vi "Configure.vi"(8 "error in (no error)":errorcluster, 11 "Retiga in":refnum<class "Retiga.lvclass">) -> (0 "error out":errorcluster, 2 "cancelled?":bool, 3 "Retiga out":refnum<class "Retiga.lvclass">)   [LabVIEW 2012, in "Retiga.lvclass"]
doc: "The configure method configures the details for the RabbitMQ connection, the observers and the mapping script.\n\nIn the derived class, make a call to the parent for setting these parameters."
uses:
  Retiga.lvclass
  <vilib>/Utility/miscctls.llb/LVPointTypeDef.ctl
  Retiga.lvclass/Retiga.ctl
  <vilib>/Distrio/Murmex/Murmex/Murmex.lvclass
panel:
  in  "button:call_parent":bool
  in  "button:cancel":bool
  in  "button:ok":bool
  in  "Tab Control":enum32{"Phase comparison", "Camera properties"}(tab)
  in  "stage component":string
  in  "micron equivalent of pixel":dbl[unit]
  in  "max x pixel displacement":dbl
  in  "max pixel discrepancy":dbl
  in  "max y pixel displacement":dbl
  in  "max physical displacement":dbl[unit]
  in  "brightness threshold":sgl
  in  "min physical displacement":dbl[unit]
  in  "temperature":dbl
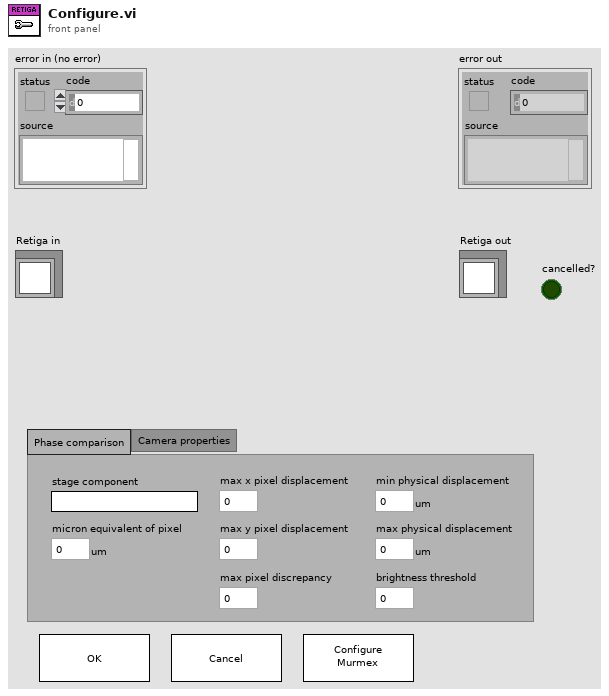
[diagram p1: front panel]
types:
  T1 = typedef "LVPointTypeDef.ctl" = cluster{"Horizontal":i16, "Vertical":i16}
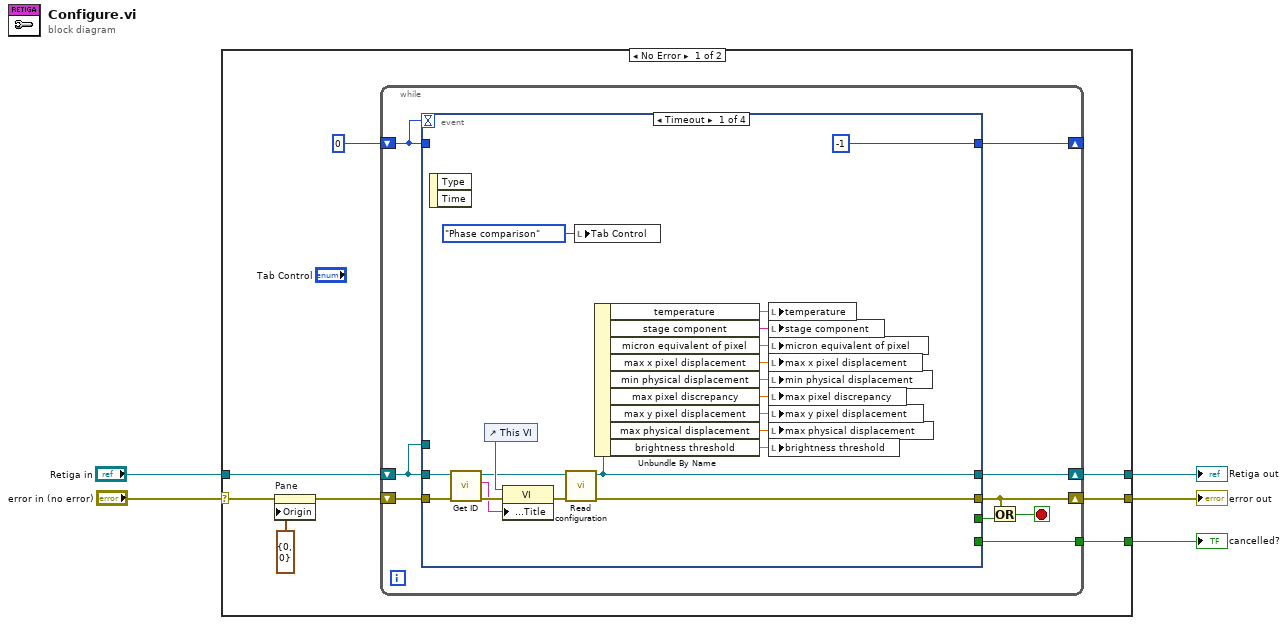
[diagram p0: block diagram]
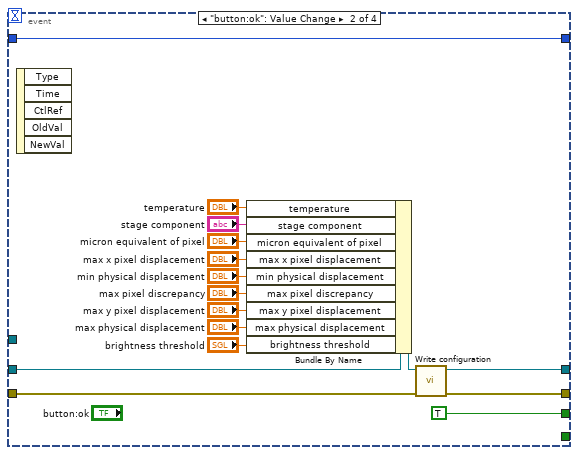
[diagram p2: hidden frame]
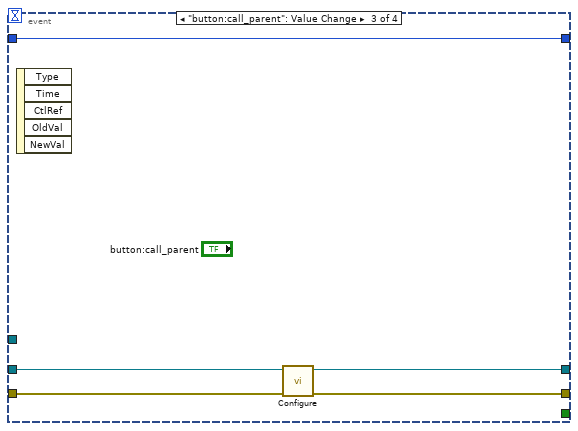
[diagram p3: hidden frame]
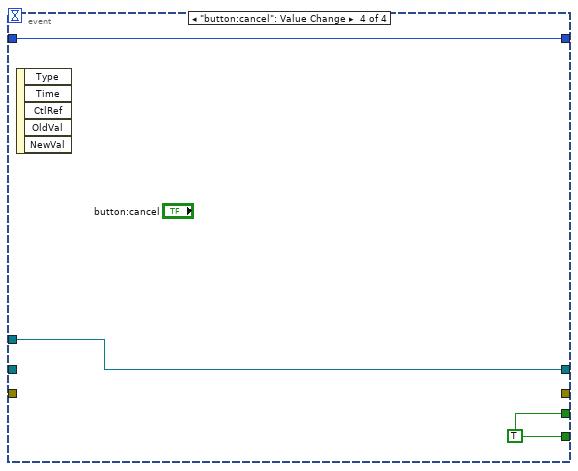
[diagram p4: hidden frame]
diagram:
  n1 = case shown="No Error" "error in (no error)" {
    selector: "error in (no error)" -> [w12 w67]
    tunnel: [w7 w68] -> w4
    tunnel: "Retiga in" -> [w10 w68]
    tunnel: [w8 w67] -> w2
    tunnel: [w6 _] -> w1
    frame No Error {
      n2 = property on="Pane" class="Pane"(error in=w12, "Origin"=T1 {"Horizontal"=0, "Vertical"=0}) -> (error out=w11:errorcluster)  [unwired: 1 in, 1 out]
      n3 = while {
        shift-right: [w16] -> w8
        shift-left: w11 -> [w22]
        shift-right: [w18] -> w7
        shift-left: w10 -> [w21]
        shift-right: [w19] -> _
        shift-left: 0 -> [w20]
        tunnel: [w14] -> w6
        stop <- w15 stop-if-true
        n4 = event shown="[0] Timeout" {
          selector: _ -> [_ _ _ _]
          dyn-events: _ -> [_ _ _ _]
          timeout: w20 -> [_ _ _ _]
          tunnel: w22 -> [w36 w58 w63 _]
          tunnel: w21 -> [w35 w56 w62 _]
          tunnel: w21 -> [_ _ _ w66]
          tunnel: w20 -> [_ w43 w59 w64]
          tunnel: [-1 w43 w59 w64] -> w19
          tunnel: [w33 w57 w60 _] -> w16
          tunnel: [w34 w54 w61 w66] -> w18
          tunnel: [_ TRUE ("y") _ w65] -> w17
          tunnel: [_ _ _ w65] -> w14
          event Timeout {
            n5 = event-data() -> ()  [unwired: 1 in, 2 out]
            n6 = call <vilib>:"Get ID.vi"("error in (no error)"=w36, "Murmex in"=w35) -> ("error out"=w41:errorcluster, "component id"=w37:string, "Murmex out"=w38:refnum<class "Retiga.lvclass">)  [unwired: 7 in]
            n7 = control-ref of="This VI"() -> (w40:refnum<vi>)
            n8 = property class="VI"(reference=w40, error in=w41, "Front Panel.Title"=w37) -> (error out=w39:errorcluster)  [unwired: 1 out]
            n9 = call <vilib>:"Read configuration.vi"("error in (no error)"=w39, "Murmex in"=w38) -> ("error out"=w33:errorcluster, "Murmex out"=w34:refnum<class "Retiga.lvclass">)  [unwired: 7 in, 1 out]
            n10 = local write "Tab Control"(enum32{"Phase comparison", "Camera properties"}."Phase comparison" ("Tab Control")) -> ()
            n11 = Unbundle By Name(w34) -> ("temperature"=w27:dbl, "stage component"=w26:string, "micron equivalent of pixel"=w28:dbl[unit], "max x pixel displacement"=w25:dbl, "min physical displacement"=w30:dbl[unit], "max pixel discrepancy"=w31:dbl, "max y pixel displacement"=w32:dbl, "max physical displacement"=w24:dbl[unit], "brightness threshold"=w29:sgl)
            n12 = local write "temperature"(w27) -> ()
            n13 = local write "stage component"(w26) -> ()
            n14 = local write "micron equivalent of pixel"(w28) -> ()
            n15 = local write "max x pixel displacement"(w25) -> ()
            n16 = local write "min physical displacement"(w30) -> ()
            n17 = local write "max pixel discrepancy"(w31) -> ()
            n18 = local write "max y pixel displacement"(w32) -> ()
            n19 = local write "max physical displacement"(w24) -> ()
            n20 = local write "brightness threshold"(w29) -> ()
          }
          event "button:ok": Value Change {
            n21 = event-data() -> ()  [unwired: 1 in, 5 out]
            n22 = Bundle By Name(cluster=w56, "temperature"="temperature", "stage component"="stage component", "micron equivalent of pixel"="micron equivalent of pixel", "max x pixel displacement"="max x pixel displacement", "min physical displacement"="min physical displacement", "max pixel discrepancy"="max pixel discrepancy", "max y pixel displacement"="max y pixel displacement", "max physical displacement"="max physical displacement", "brightness threshold"="brightness threshold") -> (w55:refnum<class "Retiga.lvclass">)
            n23 = call <vilib>:"Write configuration.vi"("error in (no error)"=w58, "Murmex in"=w55) -> ("error out"=w57:errorcluster, "Murmex out"=w54:refnum<class "Retiga.lvclass">)  [unwired: 8 in]
          }
          event "button:call_parent": Value Change {
            n24 = event-data() -> ()  [unwired: 1 in, 5 out]
            n25 = call-parent "Configure.vi"("error in (no error)"=w63, "Murmex in"=w62) -> ("error out"=w60:errorcluster, "Murmex out"=w61:refnum<class "Retiga.lvclass">)  [unwired: 7 in, 1 out]
          }
          event "button:cancel": Value Change {
            w65 = TRUE
            n26 = event-data() -> ()  [unwired: 1 in, 5 out]
          }
        }
        n27 = Or(x=w16, y=w17) -> (x .or. y?=w15:bool)
      }
    }
    frame Error {
    }
  }
  "error out" <- w2
  "Retiga out" <- w4
  "cancelled?" <- w1
